vi "AFG3352X.get i attribute.vi"(0 "i ref in":refnum<vi>, 5 "error in (no error)":errorcluster) -> (14 "i ref out":refnum<vi>, 16 "i attribute":T1={"Act2ndValues"={"frequency"=0.0, "amplitude"=0.0, "phase"=0.0, "DCOffset"=0.0, "waveformType"=enum."sine", "enableOutput"=FALSE, "trigger"=[], "serviceIDs"={"frequencyID"=0, "amplitudeID"=0, "phaseID"=0, "DCOffsetID"=0, "waveformTypeID"=0, "enableOutputID"=0, "triggerID"=0}, "waveform"={"data"={"t0"=timestamp(0 s since 1904-01-01), "dt"=0.0, "Y"=[]}, "gain"=0.0, "offset"=0.0, "repetitionRate"=0.0, "sampleRate"=0.0}}, "Nom2ndValues"={"frequency"=0.0, "amplitude"=0.0, "phase"=0.0, "DCOffset"=0.0, "waveformType"=enum."sine", "enableOutput"=FALSE, "trigger"=[], "serviceIDs"={"frequencyID"=0, "amplitudeID"=0, "phaseID"=0, "DCOffsetID"=0, "waveformTypeID"=0, "enableOutputID"=0, "triggerID"=0}, "waveform"={"data"={"t0"=timestamp(0 s since 1904-01-01), "dt"=0.0, "Y"=[]}, "gain"=0.0, "offset"=0.0, "repetitionRate"=0.0, "sampleRate"=0.0}}, "DefaultChannel"=0, "ActAddValues"={"Mode1"=0, "serviceIDs"={"Mode1ID"=0, "Mode2ID"=0, "Burst1ID"=0, "Burst2ID"=0}, "Mode2"=0, "Burst1"=1, "Burst2"=1}, "NomAddValues"={"Mode1"=0, "serviceIDs"={"Mode1ID"=0, "Mode2ID"=0, "Burst1ID"=0, "Burst2ID"=0}, "Mode2 2"=0, "Burst1"=1, "Burst2"=1}, "enableBurstMode"=FALSE} {"NomAddValues"."Burst2" items=["Triggered", "Gated"]; "NomAddValues"."Burst1" items=["Triggered", "Gated"]; "NomAddValues"."Mode2 2" items=["Normal", "Gated"]; "NomAddValues"."Mode1" items=["Normal", "Gated"]; "ActAddValues"."Burst2" items=["Triggered", "Gated"]; "ActAddValues"."Burst1" items=["Triggered", "Gated"]; "ActAddValues"."Mode2" items=["Normal", "Gated"]; "ActAddValues"."Mode1" items=["Normal", "Gated"]}, 19 "error out":errorcluster)   [LabVIEW 2014, in "AFG3352X.lvlib"]
doc: "Gets the i attribute data of an object.\n\nLicense Agreement for this software:\n\nCopyright (C)\nGesellschaft für Schwerionenforschung, GSI\nPlanckstr. 1\n64291 Darmstadt\nGermany\n\nContact: D.Beck@gsi.de \n\nThis program is free software; you can redistribute it and/or modify it under the terms of the GNU General Public License as published by the Free Software Foundation; either version 2 of the license, or (at your option) any later version.\n\nThis program is distributed in the hope that it will be useful, but WITHOUT ANY WARRANTY; without even the implied warranty of MERCHANTABILITY or FITNESS FOR A PARTICULAR PURPOSE. See the GNU General License for more details (http://www.gnu.org).\n\nGesellschaft für Schwerionenforschung, GSI\nPlanckstr. 1, 64291 Darmstadt, Germany\nFor all questions and ideas contact: M.Richter@gsi.de, H.Brand@gsi.de or D.Beck@gsi.de.\nLast update: 17-JUN-2004"
uses:
  AFG3352X.lvlib
  AFG3352X.i attribute.ctl
  CS_Core/CSApplicationBaseClasses/AFGBase/AFGBase.waveformType.ctl
  CS_Core/CSApplicationBaseClasses/AFGBase/AFGBase.lvlib
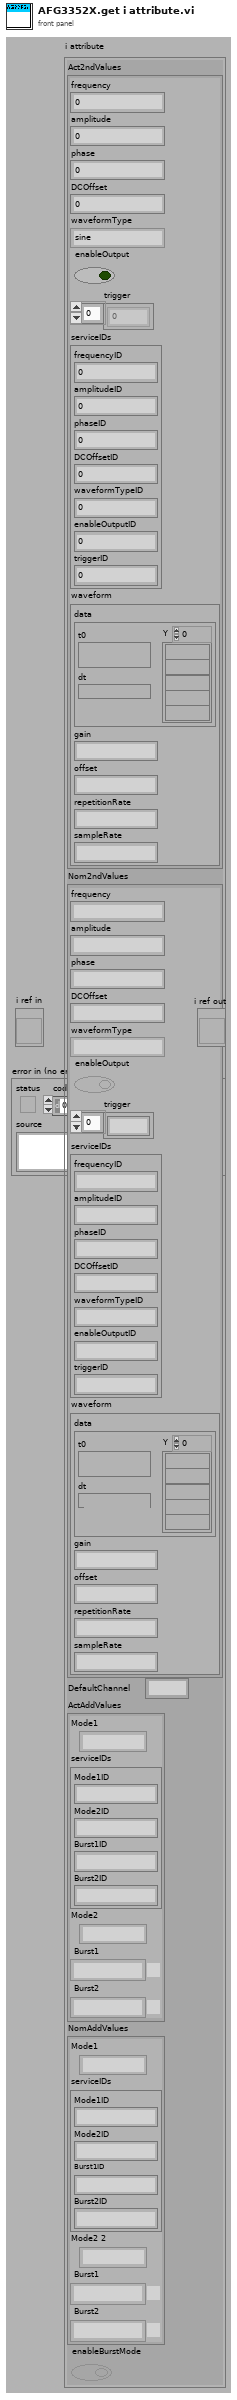
[diagram p1: front panel]
types:
  T1 = typedef "AFG3352X.lvlib/AFG3352X.i attribute.ctl" = cluster{"Act2ndValues":cluster{"frequency":dbl, "amplitude":dbl, "phase":dbl, "DCOffset":dbl, "waveformType":T2, "enableOutput":bool, "trigger":i16[], "serviceIDs":cluster{"frequencyID":i32, "amplitudeID":i32, "phaseID":i32, "DCOffsetID":i32, "waveformTypeID":i32, "enableOutputID":i32, "triggerID":i32}, "waveform":cluster{"data":waveform(dbl), "gain":dbl, "offset":dbl, "repetitionRate":dbl, "sampleRate":dbl}}, "Nom2ndValues":cluster{"frequency":dbl, "amplitude":dbl, "phase":dbl, "DCOffset":dbl, "waveformType":T2, "enableOutput":bool, "trigger":i16[], "serviceIDs":cluster{"frequencyID":i32, "amplitudeID":i32, "phaseID":i32, "DCOffsetID":i32, "waveformTypeID":i32, "enableOutputID":i32, "triggerID":i32}, "waveform":cluster{"data":waveform(dbl), "gain":dbl, "offset":dbl, "repetitionRate":dbl, "sampleRate":dbl}}, "DefaultChannel":i32, "ActAddValues":cluster{"Mode1":u16, "serviceIDs":cluster{"Mode1ID":i32, "Mode2ID":i32, "Burst1ID":i32, "Burst2ID":i32}, "Mode2":u16, "Burst1":i32, "Burst2":i32}, "NomAddValues":cluster{"Mode1":u16, "serviceIDs":cluster{"Mode1ID":i32, "Mode2ID":i32, "Burst1ID":i32, "Burst2ID":i32}, "Mode2 2":u16, "Burst1":i32, "Burst2":i32}, "enableBurstMode":bool}
  T2 = typedef "AFGBase.lvlib/AFGBase.waveformType.ctl" = enum16{"sine", "square", "ramp", "pulse", "noise", "DC", "arbitrary", "triangle", "ramp_up", "ramp_down", "amplitude modulation"}
  T3 = enum16{"SetAttribute", "GetAttribute", "CreateAttribute", "DestroyAttribute", "DestroyAllAtributes"}
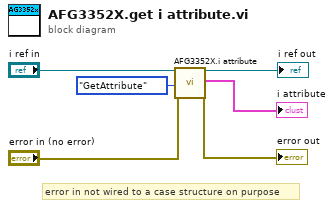
[diagram p0: block diagram]
diagram:
  # "error in not wired to a case structure on purpose"
  n1 = call "AFG3352X.i attribute.vi"("VI Refnum"="i ref in", "Action"=T3."GetAttribute", "error in (no error)"="error in (no error)") -> ("VI Refnum out"=→"i ref out":refnum<vi>, "CLASS.i attribute out"=→"i attribute":T1, "error out"=→"error out":errorcluster)  [unwired: 14 in]
